vi "Poll_Bias.vi"(8 "error in (no error)":errorcluster, 9 "Scan Parameters in":T1 {"Avoid zero threshold (V)" format="%#_13g"}, 10 "ACK Q in":refnum<queue>, 11 "Queue in":refnum<queue>) -> (0 "error out":errorcluster, 1 "Scan Parameters out":T1 {"Avoid zero threshold (V)" format="%#_13g"}, 2 "ACK Q out":refnum<queue>, 3 "Queue out":refnum<queue>)   [LabVIEW 2025]
uses:
  <userlib>/Nanonis Prog Interface V5e/Nanonis Prog Interface.lvlib
  CTLS/ACK.ctl
  CTLS/Scan_Params (QMH).ctl
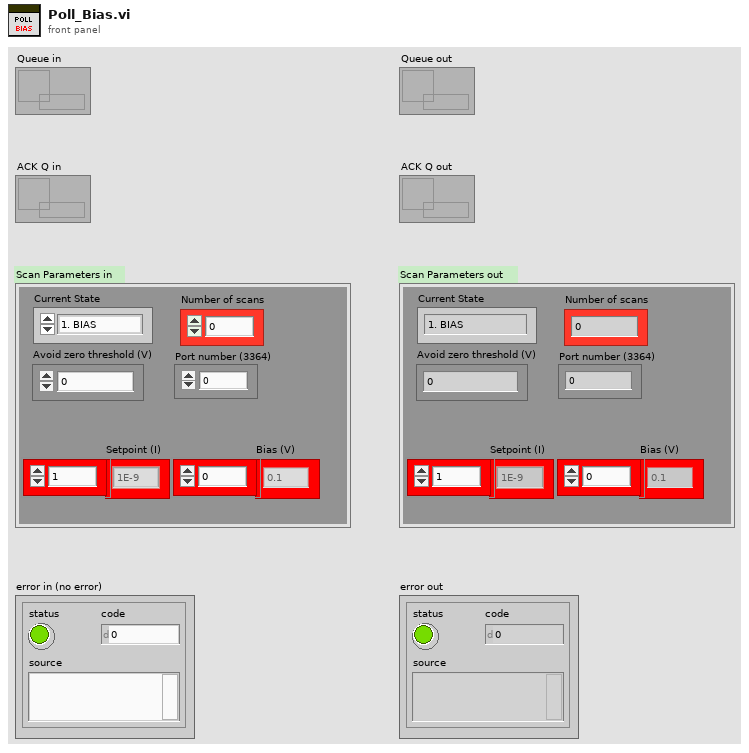
[diagram p1: front panel]
types:
  T1 = typedef "Scan_Params (QMH).ctl" = cluster{"Setpoint (I)":dbl[], "Bias (V)":dbl[], "Number of scans":u8, "Port number (3364)":u32, "Avoid zero threshold (V)":dbl, "Current State":enum16{"1. BIAS", "2. POLL BIAS", "3. SCAN", "4. SCAN_IDLE", "5. Drift_Correct (SF)", "6. Drift_Correct (BS)", "7. STOP"}}
  T2 = enum16{"1. BIAS", "2. POLL BIAS", "3. SCAN", "4. SCAN_IDLE", "5. Drift_Correct (SF)", "6. Drift_Correct (BS)", "7. STOP"}
  T3 = enum16{"1. None", "2. TempStable", "3. FieldStable", "4. ConfigApplied", "5. ScanDone", "6. BiasDone", "7. DriftDone (SF)", "8. DrifDone (BS)"}
  T4 = typedef "ACK.ctl" = cluster{"ACK":enum16{"1. None", "2. TempStable", "3. FieldStable", "4. ConfigApplied", "5. ScanDone", "6. BiasDone", "7. DriftDone (SF)", "8. DrifDone (BS)"}}
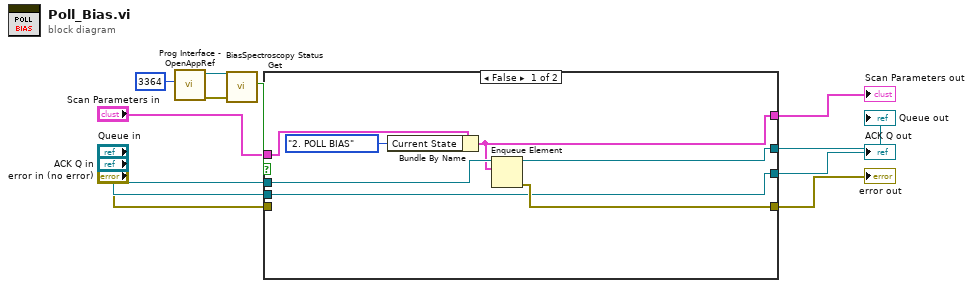
[diagram p0: block diagram]
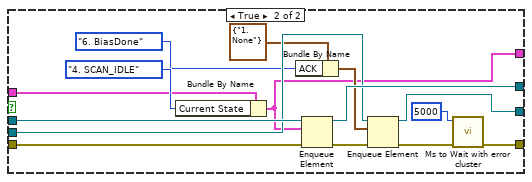
[diagram p2: hidden frame]
diagram:
  n1 = call <userlib>:"Prog Interface - OpenAppRef.vi"("Port number (3364)"=u32 3364) -> ("Error out"=w10:errorcluster, "Application reference"=w9:refnum<vi>)  [unwired: 5 in]
  n2 = call <userlib>:"BiasSpectroscopy Status Get.vi"("Error in (no error)"=w10, "Application ref in"=w9) -> ("Running?"=w11:bool)  [unwired: 5 in, 2 out]
  n3 = case shown="False" w11 {
    tunnel: "Queue in" -> [w19 w34]
    tunnel: [w16 w33] -> w2
    tunnel: "error in (no error)" -> [_ w32]
    tunnel: "ACK Q in" -> [w14 w30]
    tunnel: [w14 w27] -> w5
    tunnel: "Scan Parameters in" -> [w18 w24]
    tunnel: [w13 w23] -> w7
    tunnel: [w15 w21] -> w8
    frame False {
      n4 = Bundle By Name(cluster=w18, "Current State"=T2."2. POLL BIAS") -> (w13:T1)
      n5 = Enqueue Element(queue=w19, element=w13) -> (queue out=w16:refnum<queue>, error out=w15:errorcluster)  [unwired: 2 in, 1 out]
    }
    frame True {
      n6 = Bundle By Name(cluster=w24, "Current State"=T2."4. SCAN_IDLE") -> (w23:T1)
      n7 = Bundle By Name(cluster=T4 {"ACK"=enum."1. None"} ("Acknowledements"), "ACK"=T3."6. BiasDone") -> (w28:T4)
      n8 = Enqueue Element(queue=w34, element=w23, error in (no error)=w32) -> (queue out=w33:refnum<queue>, error out=w26:errorcluster)  [unwired: 1 in, 1 out]
      n9 = Enqueue Element(queue=w30, element=w28, error in (no error)=w26) -> (queue out=w27:refnum<queue>, error out=w22:errorcluster)  [unwired: 1 in, 1 out]
      n10 = call <userlib>:"Ms to Wait with error cluster.vi"("error in (no error)"=w22, "milliseconds to wait"=u32 5000) -> ("error out"=w21:errorcluster)  [unwired: 4 in, 1 out]
    }
  }
  "error out" <- w8
  "Scan Parameters out" <- w7
  "ACK Q out" <- w5
  "Queue out" <- w2
